vi "GlobalStatus.vi"() -> ()   [LabVIEW 2012]
panel:
  out "hangar full":bool
  out "too many flies":bool
  in  "program status":T1(ring)
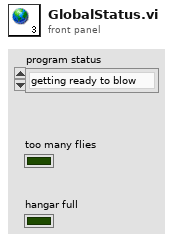
[diagram p1: front panel]
types:
  T1 = enum16{"getting ready to blow", "blowing the fly", "waiting for fly"}
diagram:
